vi "Calibrate.vi"(8 "error in (no error)":errorcluster, 10 "Calibration Type (0: All)":i32(ring) items=["All", "Flatness for AC Path"], 11 "VISA resource name":refnum<visa-resource-name>) -> (0 "error out":errorcluster, 2 "Pass/Fail":bool, 3 "VISA resource name out":refnum<visa-resource-name>)   [LabVIEW 2020, in "Agilent 34405.lvlib"]
doc: "Performs a calibration of the multimeter using the specified calibration value.\n\n<B>Notes:</B>\n(1) Before you can calibrate the instrument, you must unsecure it by entering the correct security code."
uses:
  <instrlib>/Agilent 34405/Agilent 34405.lvlib
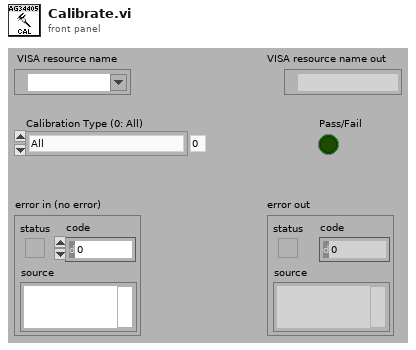
[diagram p1: front panel]
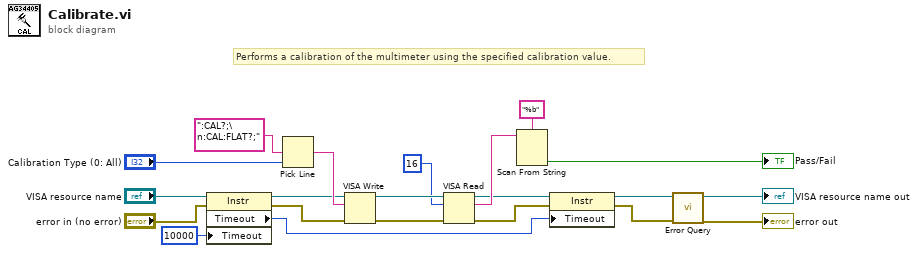
[diagram p0: block diagram]
diagram:
  # "Performs a calibration of the multimeter using the specified calibration value."
  n1 = property on="Property Node" class="Instr"(reference="VISA resource name", error in="error in (no error)", "Timeout"=u32 10000 ("General Settings:Timeout Value")) -> (reference out=w7:refnum<visa-resource-name>, error out=w6:errorcluster, "Timeout"=w3:u32)
  n2 = Pick Line(multi-line string=":CAL?;\n:CAL:FLAT?;", line index="Calibration Type (0: All)") -> (output string=w11:string)  [unwired: 1 out]
  n3 = VISA Write(VISA resource name=w7, write buffer=w11, error in (no error)=w6) -> (VISA resource name out=w19:refnum<visa-resource-name>, error out=w18:errorcluster)  [unwired: 1 out]
  n4 = VISA Read(VISA resource name=w19, byte count=u32 16, error in (no error)=w18) -> (VISA resource name out=w5:refnum<visa-resource-name>, read buffer=w16:string, error out=w4:errorcluster)  [unwired: 1 out]
  n5 = Scan From String(format string="%b", input string=w16) -> (output 1=→"Pass/Fail":bool)  [unwired: 2 in, 4 out]
  n6 = property on="Property Node" class="Instr"(reference=w5, error in=w4, "Timeout"=w3) -> (reference out=w2:refnum<visa-resource-name>, error out=w1:errorcluster)
  n7 = call <instrlib>:"Error Query.vi"("error in (no error)"=w1, "VISA resource name"=w2) -> ("error out"=→"error out":errorcluster, "VISA resource name out"=→"VISA resource name out":refnum<visa-resource-name>)  [unwired: 8 out]
